vi "cw_3_5.vi"() -> ()   [LabVIEW 2022 SP3]
panel:
  out "Array":i32[](array[numeric])
  in  "M":i32
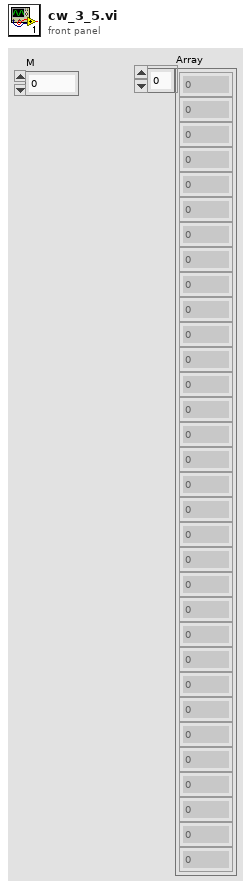
[diagram p1: front panel]
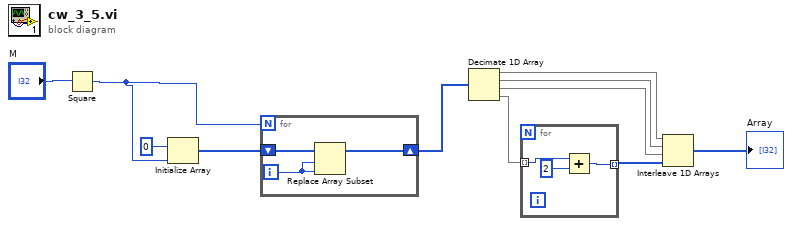
[diagram p0: block diagram]
diagram:
  n1 = Square(x="M") -> (x^2=w5:i32)
  n2 = Initialize Array(0 ("element"), w5) -> (w10:i32[])
  n3 = for {
    N: w5 -> [_]
    shift-right: [w12] -> w6
    shift-left: w10 -> [w14]
    i -> [w13]
    n4 = Replace Array Subset(array=w14, new element=w13, index=w13) -> (w12:i32[])
  }
  n5 = Decimate 1D Array(w6) -> (w1:i32[], w2:i32[], w3:i32[], w8:i32[])
  n6 = for {
    tunnel: w8 -> [w17] mode=indexing
    tunnel: [w15] -> w4 mode=indexing
    n7 = Add(x=w17, y=2) -> (x+y=w15:i32)
  }
  n8 = Interleave 1D Arrays(w1, w2, w3, w4) -> (→"Array":i32[])
